vi "Blue Team Data.vi"() -> ()   [LabVIEW 2018]
panel:
  out "B Triangle":T1
  out "B Square":T1
  out "B Circle":T1
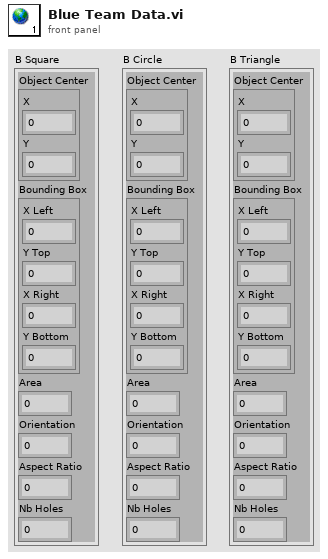
[diagram p1: front panel]
types:
  T1 = cluster{"Object Center":cluster{"X":sgl, "Y":sgl}, "Bounding Box":cluster{"X Left":i32, "Y Top":i32, "X Right":i32, "Y Bottom":i32}, "Area":sgl, "Orientation":sgl, "Aspect Ratio":sgl, "Nb Holes":i32}
diagram:
